vi "Get Default for Type.vi"(8 "error in (no error)":errorcluster, 11 "Path of Type":path) -> (0 "error out":errorcluster, 3 "Default for Type":variant)   [LabVIEW 2020, in "MeasurementLink Measurement Server.lvlib"]
uses:
  MeasurementLink Measurement Server.lvlib
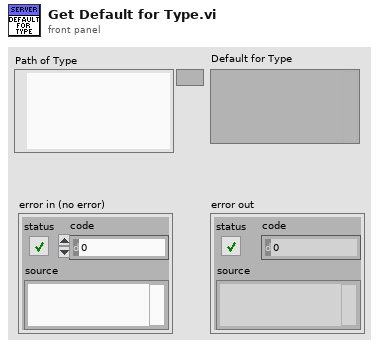
[diagram p1: front panel]
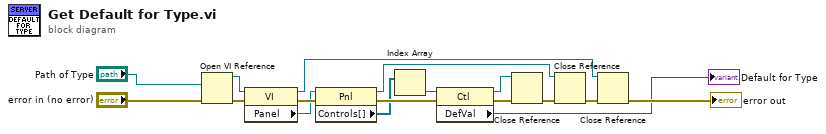
[diagram p0: block diagram]
diagram:
  n1 = Open VI Reference(vi path="Path of Type", error in (no error)="error in (no error)") -> (vi reference=w5:refnum<vi>, error out=w14:errorcluster)  [unwired: 4 in]
  n2 = property class="VI"(reference=w5, error in=w14) -> (reference out=w10:refnum<vi>, error out=w13:errorcluster, "Panel"=w6:refnum<vi>)
  n3 = property class="Pnl"(reference=w6, error in=w13) -> (reference out=w9:refnum<vi>, error out=w15:errorcluster, "Controls[]"=w7:refnum<vi>[])
  n4 = Index Array(array=w7) -> (element=w16:refnum<vi>)  [unwired: 1 in]
  n5 = property class="Ctl"(reference=w16, error in=w15) -> (reference out=w8:refnum<vi>, error out=w17:errorcluster, "DefVal"=→"Default for Type":variant)
  n6 = Close Reference(reference=w8, error in (no error)=w17) -> (error out=w12:errorcluster)
  n7 = Close Reference(reference=w9, error in (no error)=w12) -> (error out=w11:errorcluster)
  n8 = Close Reference(reference=w10, error in (no error)=w11) -> (error out=→"error out":errorcluster)
